vi "MultiOpto_Begin.vi"() -> (0 "NI DMM 2 Status":bool, 1 "NI DMM 1 Status":bool, 2 "Ophir 2 Status":bool, 3 "Ophir 1 Status":bool, 4 "Текущий Образец №":string, 5 "NI Scope Status":bool, 8 "NI DMM 2 option return":enum32{"Ampermeter button", "Ohmmeter button"}(ring), 9 "NI DMM 1 option return":enum32{"Ampermeter button", "Ohmmeter button"}(ring))   [LabVIEW 2018]
panel:
  in  "NI DMM 2 option":enum32{"Ampermeter button", "Ohmmeter button"}(radio)
  in  "NI DMM 1 option":enum32{"Ampermeter button", "Ohmmeter button"}(radio)
  in  "Ophir 2":bool
  in  "NI DMM 2":bool
  out "Boolean 4":bool
  out "Boolean 3":bool
  in  "Ophir 1":bool
  in  "NI DMM 1":bool
  in  "NI Scope":bool
  in  "Образец №":string
  in  "Подтвердить":bool
  out "Boolean":bool
  out "Boolean 2":bool
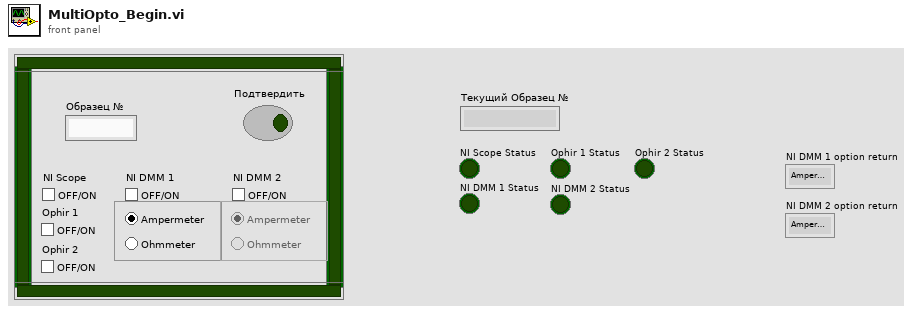
[diagram p1: front panel]
types:
  T1 = enum8{"Enabled", "Disabled", "Disabled and Grayed Out"}
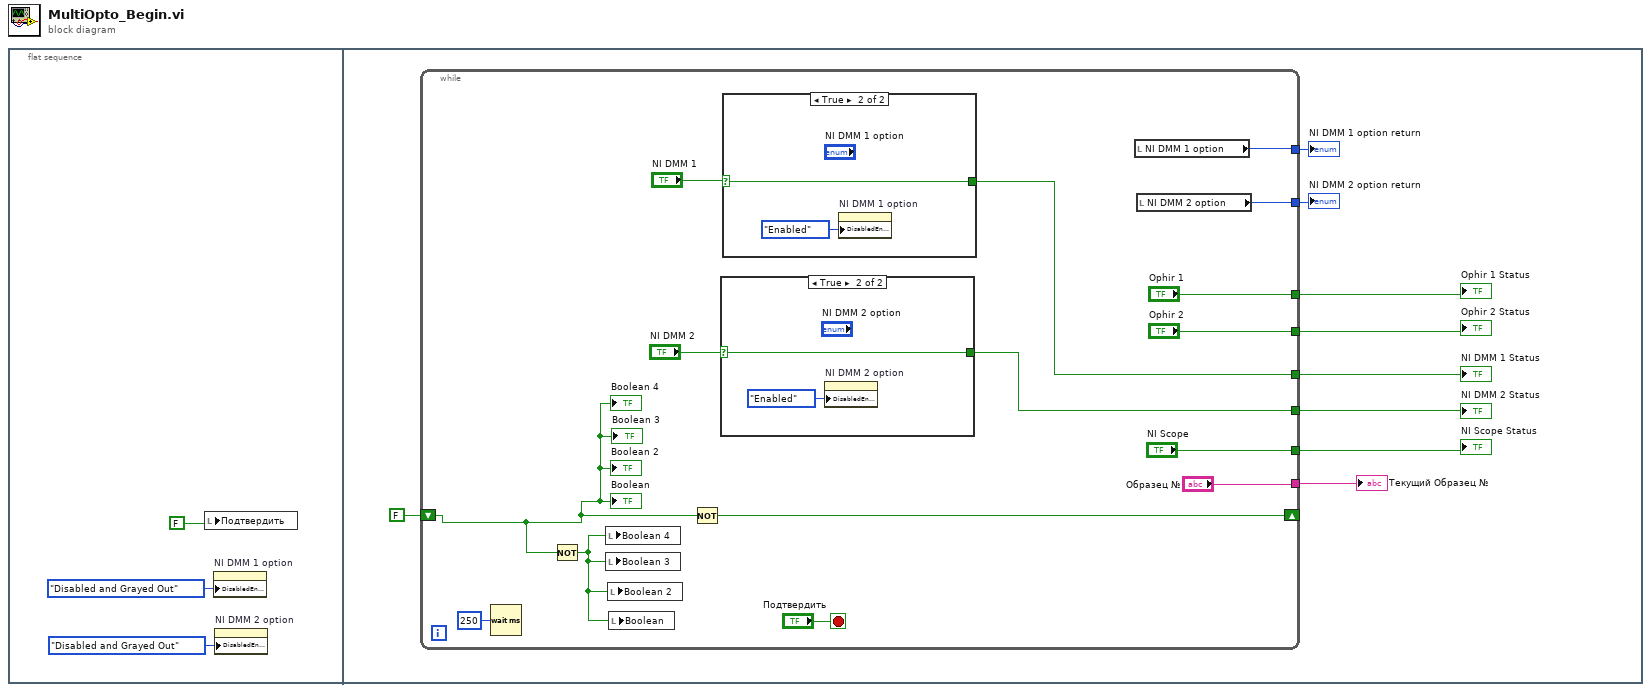
[diagram p0: block diagram]
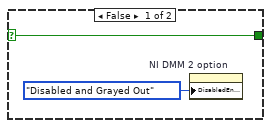
[diagram p2: hidden frame]
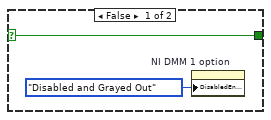
[diagram p3: hidden frame]
diagram:
  n1 = flat-sequence {
    frame #0 {
      n2 = local write "Подтвердить"(FALSE ("Ввел!")) -> ()
      n3 = property on="NI DMM 1 option" class="RadioBtnsControl (strict)"("DisabledEnum"=T1."Disabled and Grayed Out" ("Disabled")) -> ()  [unwired: 2 in, 2 out]
      n4 = property on="NI DMM 2 option" class="RadioBtnsControl (strict)"("DisabledEnum"=T1."Disabled and Grayed Out" ("Disabled")) -> ()  [unwired: 2 in, 2 out]
    }
    frame #1 {
      n5 = while {
        tunnel: ["Образец №"] -> w12
        shift-right: [w24] -> _
        shift-left: FALSE -> [w23]
        tunnel: ["NI Scope"] -> w10
        tunnel: [w16] -> w9
        tunnel: ["Ophir 1"] -> w8
        tunnel: [w15] -> w7
        tunnel: ["Ophir 2"] -> w6
        tunnel: [w14] -> w5
        tunnel: [w13] -> w4
        stop <- "Подтвердить" stop-if-true
        n6 = Wait (ms)(milliseconds to wait=u32 250) -> ()  [unwired: 1 out]
        n7 = Not(x=w23) -> (.not. x?=w22:bool)
        n8 = local write "Boolean 4"(w22) -> ()
        n9 = local write "Boolean 3"(w22) -> ()
        n10 = local write "Boolean 2"(w22) -> ()
        n11 = local write "Boolean"(w22) -> ()
        n12 = Not(x=w23) -> (.not. x?=w24:bool)
        n13 = case shown="True" "NI DMM 2" {
          selector: "NI DMM 2" -> [w28 w31]
          tunnel: [w28 w31] -> w15
          frame False {
            n14 = property on="NI DMM 2 option" class="RadioBtnsControl (strict)"("DisabledEnum"=T1."Disabled and Grayed Out" ("Disabled")) -> ()  [unwired: 2 in, 2 out]
          }
          frame True {
            n15 = property on="NI DMM 2 option" class="RadioBtnsControl (strict)"("DisabledEnum"=T1."Enabled" ("Disabled")) -> ()  [unwired: 2 in, 2 out]
          }
        }
        n16 = case shown="True" "NI DMM 1" {
          selector: "NI DMM 1" -> [w32 w35]
          tunnel: [w32 w35] -> w16
          frame False {
            n17 = property on="NI DMM 1 option" class="RadioBtnsControl (strict)"("DisabledEnum"=T1."Disabled and Grayed Out" ("Disabled")) -> ()  [unwired: 2 in, 2 out]
          }
          frame True {
            n18 = property on="NI DMM 1 option" class="RadioBtnsControl (strict)"("DisabledEnum"=T1."Enabled" ("Disabled")) -> ()  [unwired: 2 in, 2 out]
          }
        }
        n19 = local read "NI DMM 1 option"() -> (w14:enum32{"Ampermeter button", "Ohmmeter button"})
        n20 = local read "NI DMM 2 option"() -> (w13:enum32{"Ampermeter button", "Ohmmeter button"})
        "Boolean" <- w23
        "Boolean 2" <- w23
        "Boolean 3" <- w23
        "Boolean 4" <- w23
      }
      "Текущий Образец №" <- w12
      "NI Scope Status" <- w10
      "NI DMM 1 Status" <- w9
      "Ophir 1 Status" <- w8
      "NI DMM 2 Status" <- w7
      "Ophir 2 Status" <- w6
      "NI DMM 2 option return" <- w4
      "NI DMM 1 option return" <- w5
    }
  }
